vi "Configuration Utility.vi"() -> ()   [LabVIEW 2013, in "configuration library.lvlib"]
doc: "This is the main VI for the configuration editor."
uses:
  configuration library.lvlib
  Controls/StateCluster.ctl
  <vilib>/NI/Tag Bus Data Framework/Configuration Editor/Classes/SystemConfigRepo/SystemConfigRepo.lvclass
  <vilib>/NI/Configuration Framework/Node/NodeRef.ctl
  <vilib>/NI/Configuration Framework/Node/NISE_CEF_Node.lvclass
  subVI/SplashScreen/splash screen.ctl
  subVI/SplashScreen/notifier data.ctl
  <vilib>/NI/Configuration Framework/Node/StandardEvents.ctl
  <vilib>/NI/Configuration Framework/Node/UserEventRef.ctl
  <vilib>/NI/Configuration Framework/Controls/EventCluster.ctl
  <vilib>/NI/Configuration Framework/Node/NodeChangeEvent.ctl
  <vilib>/NI/Configuration Framework/Node/CacheState.ctl
  <vilib>/NI/Configuration Framework/Node/RefreshUIEvent.ctl
  <vilib>/NI/Configuration Framework/Node/StopEvent.ctl
  <vilib>/NI/Configuration Framework/glyph manager/glyph manager.ctl
  <vilib>/picture/picture.llb/imagedata.ctl
  Controls/add message.ctl
  Controls/MoveMessage.ctl
  <vilib>/NI/Tag Bus Data Framework/Configuration Editor/Classes/Systems/Systems.lvclass
  <vilib>/NI/Configuration Framework/Repository/NISE_CEF_Repository.lvclass
  <vilib>/NI/AMC/Create Single Message.vi
  <vilib>/NI/AMC/Update Message Routing Info.vi
  <vilib>/NI/AMC/Read Termination Message.vi
  <vilib>/NI/Tag Bus Data Framework/Configuration Editor/subVIs/Glyphs Status.ctl
  <vilib>/NI/Tag Bus Data Framework/Configuration Editor/subVIs/Add status to name.vi
  <vilib>/NI/AMC/Send Message.vi
  <vilib>/NI/AMC/Globals.vi
  <vilib>/NI/Tag Bus Data Framework/Configuration Editor/Classes/Module editor node/module editor node.lvclass
  <vilib>/NI/Tag Bus Data Framework/Configuration Editor/Classes/EngineTags/EngineTags.lvclass
  <vilib>/NI/Module Timing Source/timing source/TBM timing source.lvclass
  <vilib>/NI/Tag Bus Data Framework/Configuration Editor/Classes/TBM Configuration Node/TBM Configuration Node.lvclass
  <vilib>/NI/Tag Bus Module Framework/root configuration/TBM configuration.lvclass
  <vilib>/NI/Tag Bus Data Framework/Framework Configuration Classes/target configuration/PL_Target Configuration.lvclass
  <vilib>/NI/Tag Bus Data Framework/Configuration Editor/Classes/Targets/Targets.lvclass
  <vilib>/NI/Tag Bus Data Framework/Configuration Editor/Classes/Engine Parent/Engine Parent Editor Node.lvclass
  <vilib>/NI/Tag Bus Data Framework/Framework Configuration Classes/system configuration/PL_System Configuration.lvclass
  <vilib>/NI/Module Execution Interface/Engine Configuration/engine configuration.lvclass
  <vilib>/NI/Tag Bus Module Framework/channel/TBM channel.lvclass
  <vilib>/NI/Tag Bus Module Framework/module configuration/TBM module configuration.lvclass
  <vilib>/NI/AMC/AMC.lvlib
  <vilib>/NI/Configuration Framework/NISE_CEF_TreeControl.lvlib
  subVI/SplashScreen/splash screen.lvlib
  <vilib>/NI/Tag Bus Data Framework/Framework Configuration Classes/class cache/PL_class cache.lvlib
  <vilib>/NI/Tag Bus Data Framework/Configuration Editor/PL Framework Configuration Tool.lvlib
  <vilib>/NI/Configuration Framework/hierarchy repo/NISE_CEF_HierarchyRepo.lvclass
  <vilib>/NI/Configuration Framework/tree serializer/NISE_CEF_TreeSerializer.lvlib
  <vilib>/NI/Configuration Framework/glyph manager/glyph manager.lvlib
panel:
  in  "Exit":bool
  in  "View":string(tree)
  # "Tag Bus Configuration Editor"
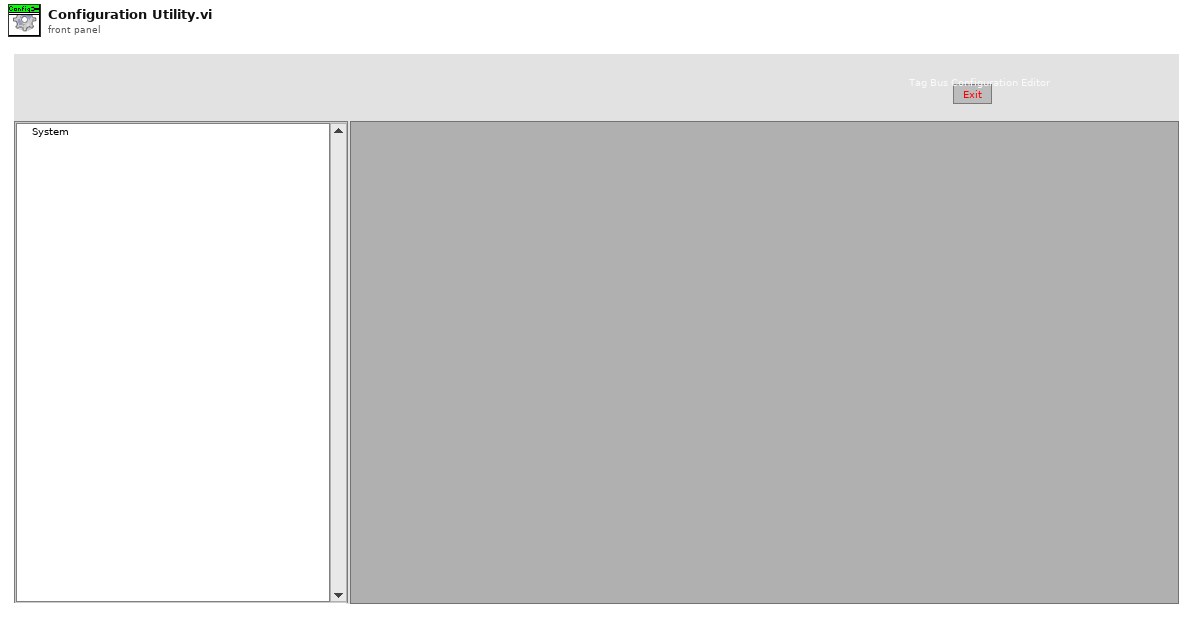
[diagram p1: front panel]
types:
  T1 = enum32{"Invalid", "Standard", "Closed", "Hidden", "Minimized", "Maximized"}
  T2 = typedef "configuration library.lvlib/StateCluster.ctl" = cluster{"repository":refnum<class "SystemConfigRepo.lvclass">, "root":T3, "unsaved changes":bool, "current path":path, "SplashScreen":T4, "classes cache":path, "standard events":T5, "glyph manager":T11}
  T3 = typedef "NISE_CEF_Node.lvclass/NodeRef.ctl" = refnum<data-value>
  T4 = typedef "configuration library.lvlib/splash screen.lvlib/splash screen.ctl" = cluster{"reference":refnum<vi>, "update notifier":refnum<notifier>, "Initialized":bool}
  T5 = typedef "NISE_CEF_Node.lvclass/StandardEvents.ctl" = cluster{"user event":T6, "node change":T7, "cache state":T8, "refresh UI":T9, "stop event":T10}
  T6 = typedef "NISE_CEF_Node.lvclass/UserEventRef.ctl" = refnum<user-event>
  T7 = typedef "NISE_CEF_Node.lvclass/NodeChangeEvent.ctl" = refnum<user-event>
  T8 = typedef "NISE_CEF_Node.lvclass/CacheState.ctl" = refnum<user-event>
  T9 = typedef "NISE_CEF_Node.lvclass/RefreshUIEvent.ctl" = refnum<user-event>
  T10 = typedef "NISE_CEF_Node.lvclass/StopEvent.ctl" = refnum<user-event>
  T11 = typedef "glyph manager.lvlib/glyph manager.ctl" = cluster{"search paths":path[], "glyph map":variant, "base glyphs":T12[], "desired overlays":string[]}
  T12 = typedef "imagedata.ctl" = cluster{"image type":i32, "image depth":i32, "image":u8[], "mask":u8[], "colors":u32[], "Rectangle":cluster{"left":i16, "top":i16, "right":i16, "bottom":i16}}
  T13 = typedef "AMC.lvlib/Message Queue.ctl" = refnum<queue>
  T14 = typedef "configuration library.lvlib/splash screen.lvlib/notifier data.ctl" = cluster{"Text":string, "percent":dbl}
  T15 = cluster{"node id":string, "RightClickPath":string}
  T16 = typedef "configuration library.lvlib/add message.ctl" = cluster{"node type":string, "to add to":string}
  T17 = typedef "configuration library.lvlib/MoveMessage.ctl" = cluster{"node ref":T3, "new parent":T3}
  T18 = typedef "configuration library.lvlib/FilePaths.ctl" = cluster{"glyphs":path[], "classes":path, "classes cache":path}
  T19 = typedef "PL_class cache.lvlib/cache definition.ctl" = cluster{"configuration":T20, "class cache data":T21}
  T20 = typedef "PL_class cache.lvlib/cache search configuration.ctl" = cluster{"Search Paths":path[], "Folders to Exclude":string[], "full class list":path[]}
  T21 = typedef "PL_class cache.lvlib/cached class information.ctl" = cluster{"targets":T22[], "engines":T23[], "modules":T23[], "ignored class list":path[]}
  T22 = typedef "PL_class cache.lvlib/target class metadata.ctl" = cluster{"file name":string, "fully qualified name":string, "menu display name":string, "configuration class name":string}
  T23 = typedef "PL_class cache.lvlib/class metadata.ctl" = cluster{"file name":string, "fully qualified name":string, "menu display name":string, "configuration class":string, "instances allowed":i32, "supported targets":T24[]}
  T24 = typedef "TBM configuration.lvclass/Target Types.ctl" = enum16{"Windows", "Mac", "Linux", "Linux RT ARM", "VxWorks", "Pharlap", "Other", "Linux RT x64"}
  T25 = typedef "NISE_CEF_Node.lvclass/Summary.ctl" = cluster{"ID":string, "parent ID":string, "node type":string, "text":string, "additional text":string, "glyph":string, "depth":i32, "glyph overlay":string}
  T26 = typedef "LVPoint32TypeDef.ctl" = cluster{"Horizontal":i32, "Vertical":i32}
  T27 = cluster{"data name":string, "drag data":variant}[]
  T28 = typedef "NISE_CEF_Node.lvclass/NodeMenuOptions.ctl" = cluster{"removable":bool, "movable":bool, "duplicate":bool}
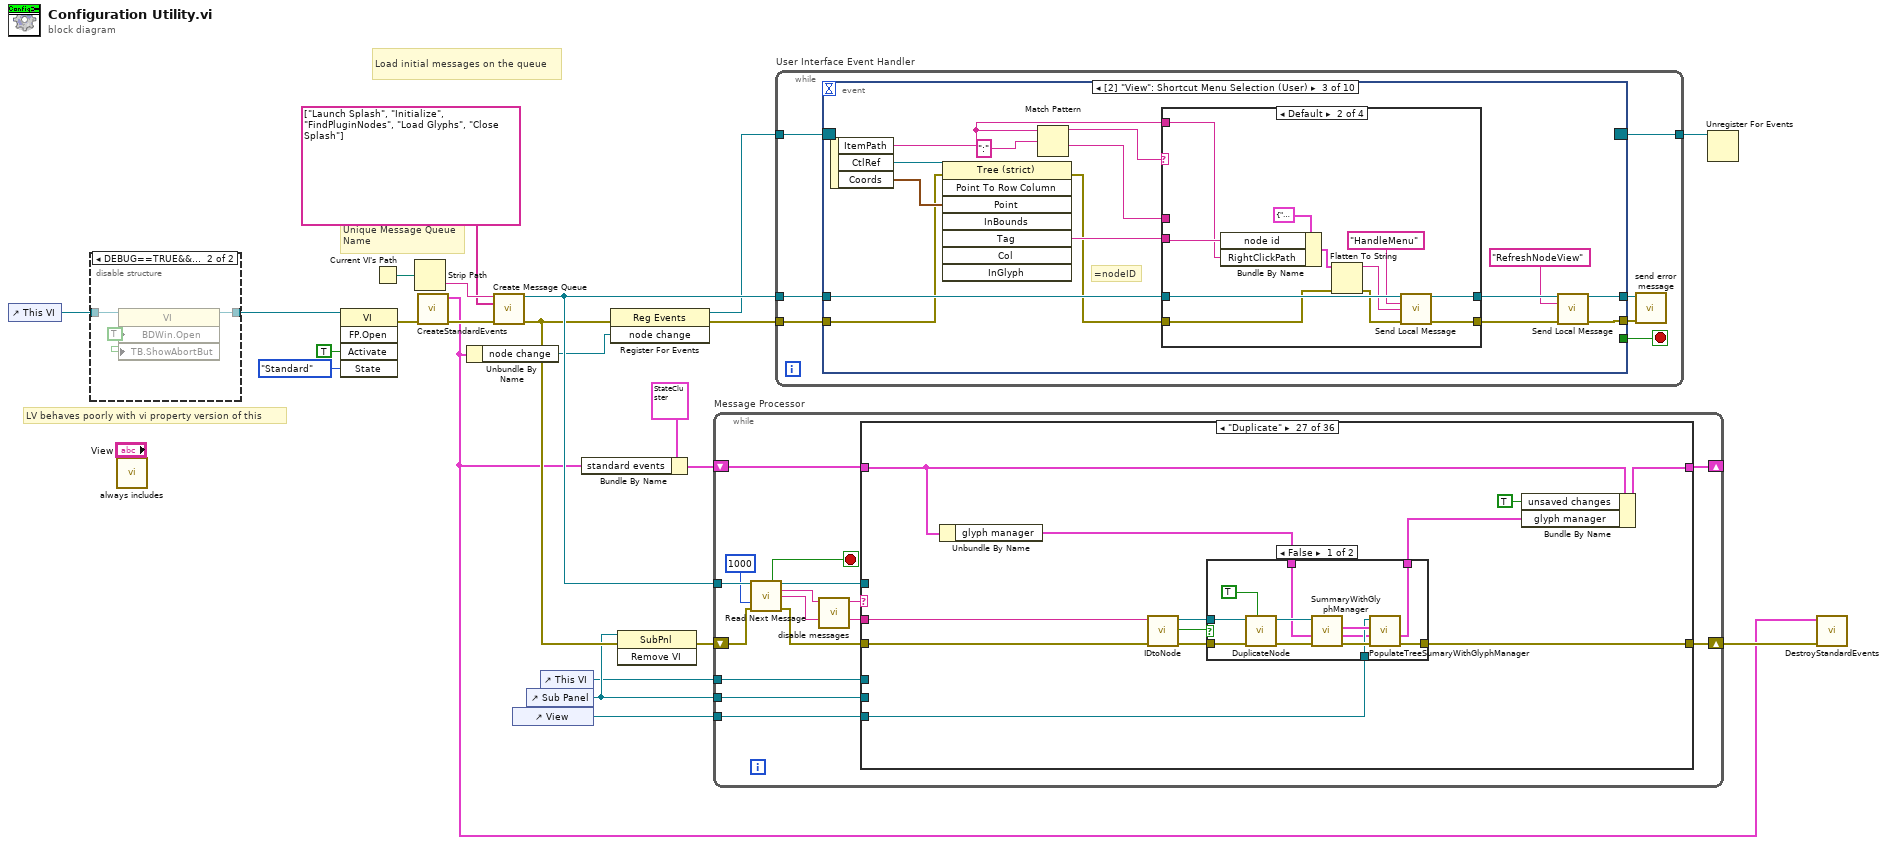
[diagram p0: block diagram]
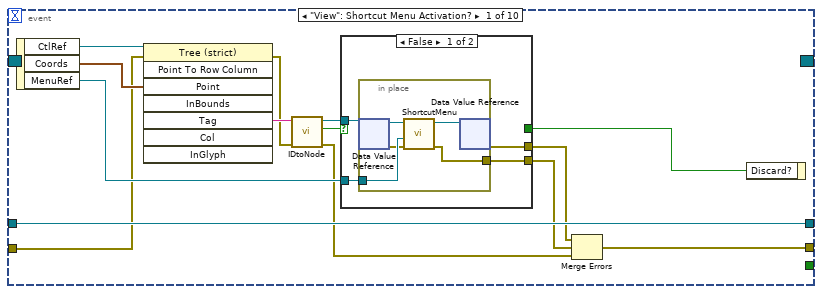
[diagram p3: hidden frame]
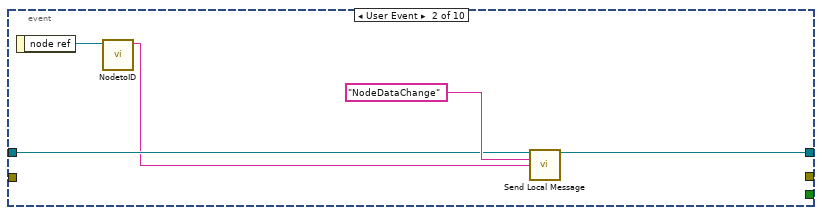
[diagram p5: hidden frame]
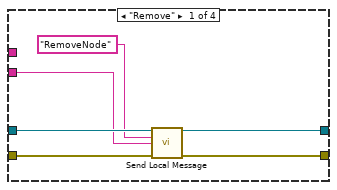
[diagram p6: hidden frame]
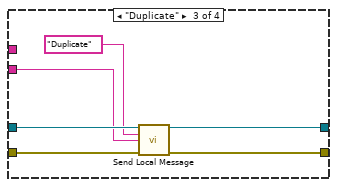
[diagram p7: hidden frame]
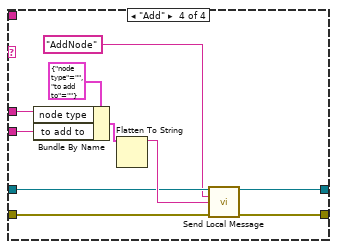
[diagram p8: hidden frame]
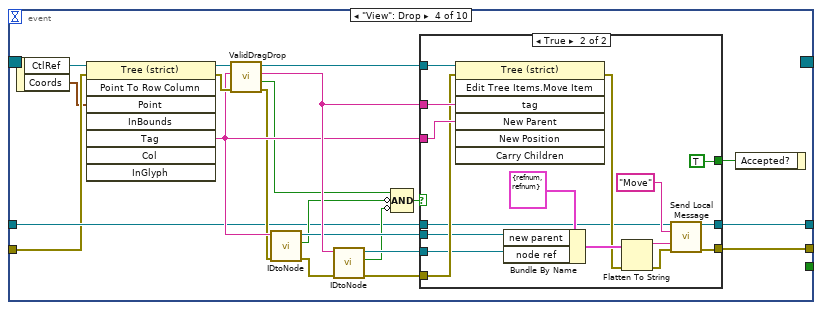
[diagram p9: hidden frame]
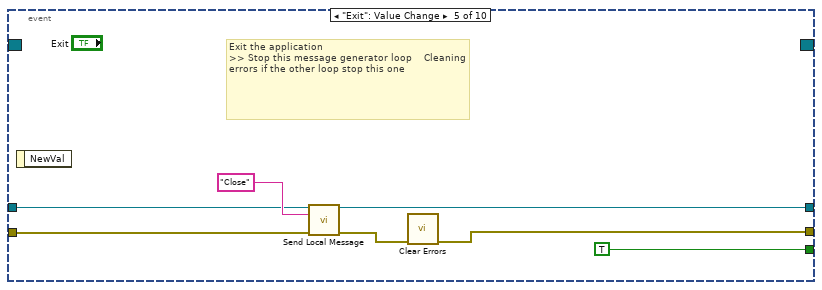
[diagram p11: hidden frame]
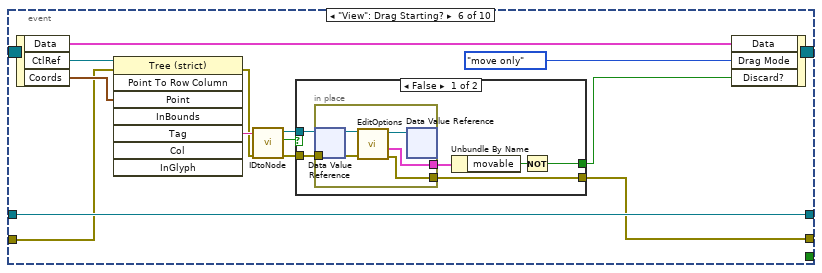
[diagram p12: hidden frame]
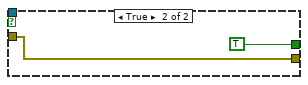
[diagram p13: hidden frame]
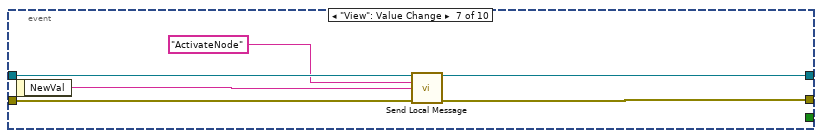
[diagram p14: hidden frame]
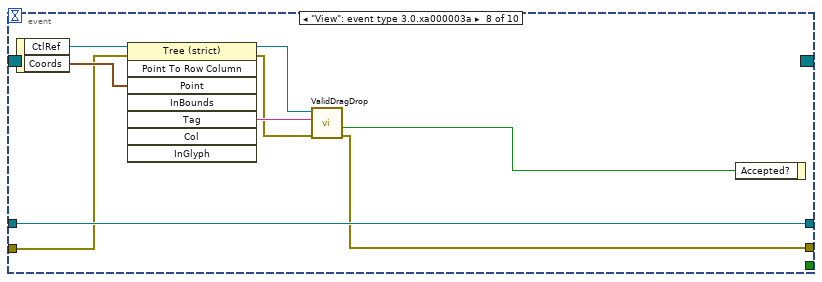
[diagram p15: hidden frame]
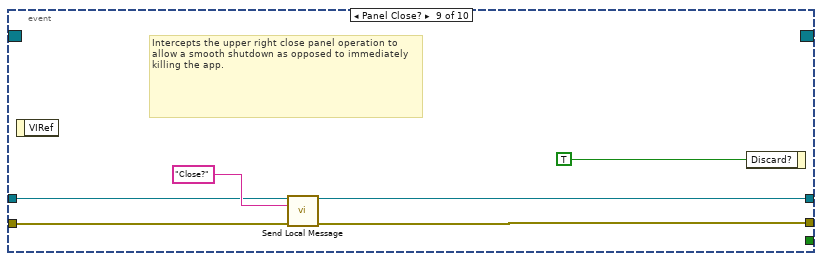
[diagram p16: hidden frame]
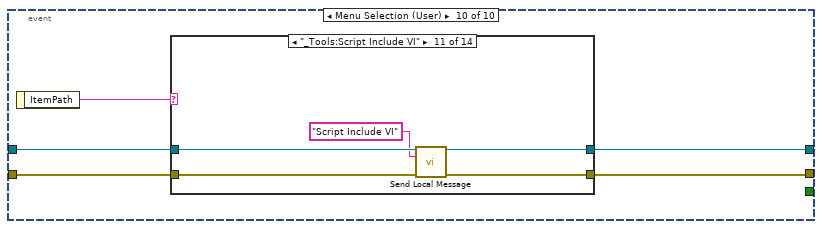
[diagram p17: hidden frame]
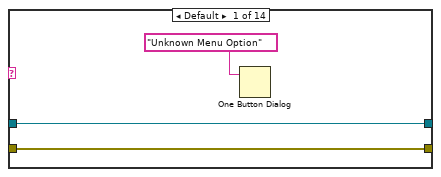
[diagram p18: hidden frame]
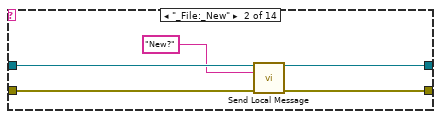
[diagram p19: hidden frame]
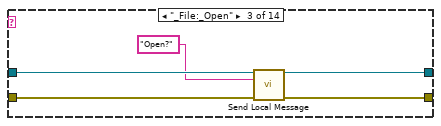
[diagram p20: hidden frame]
diagram:
  # "LV behaves poorly with vi property version of this"
  # "Unique Message Queue Name"
  # "Load initial messages on the queue"
  n1 = control-ref of="This VI"() -> (w14:refnum<vi>)
  n2 = disable-structure shown="DEBUG==TRUE&&RUN_TIME_ENGINE==False" {
    disable-tunnel: [w24 w27] -> w15
    disable-tunnel: w14 -> [w24 w26]
    frame condition #0 (active) {
    }
    frame condition #1 {
      w25 = TRUE ("Block Diagram Window:Open")
      n3 = property class="VI"(reference=w26, "BDWin.Open"=w25, "TB.ShowAbortBut"=w25) -> (reference out=w27:refnum<vi>)  [unwired: 1 in, 1 out]
    }
  }
  n4 = call "always includes.vi"() -> ()  [unwired: 12 in]
  n5 = invoke class="VI" method="FP.Open"(reference=w15, "Activate"=TRUE ("Activate?"), "State"=T1."Standard") -> (error out=w9:errorcluster)  [unwired: 2 in, 4 out]
  n6 = Current VI's Path() -> (path=w22:path)
  n7 = Strip Path(path=w22) -> (name=w23:string)  [unwired: 1 out]
  n8 = call <vilib>:"CreateStandardEvents.vi"("error in"=w9) -> ("error out"=w8:errorcluster, "standard events"=w1:T5)  [unwired: 9 in]
  n9 = Unbundle By Name(w1) -> ("node change"=w6:T7)
  n10 = call <vilib>:"Create Message Queue.vi"("message queue name"=w23, "initial message names"=string[] ["Launch Splash", "Initialize", "FindPluginNodes", "Load Glyphs", "Close Splash"], "error in"=w8) -> ("message queue out"=w20:T13, "error out"=w18:errorcluster)  [unwired: 11 in]
  n11 = control-ref of="View"() -> (w13:refnum<vi>)
  n12 = control-ref of="Sub Panel"() -> (w11:refnum<vi>)
  n13 = control-ref of="This VI"() -> (w10:refnum<vi>)
  n14 = Bundle By Name(cluster=T2 {"repository"=refnum, "root"=refnum, "unsaved changes"=FALSE, "current path"=path "", "SplashScreen"={"reference"=refnum, "update notifier"=refnum, "Initialized"=FALSE}, "classes cache"=path "", "standard events"={"user event"=refnum, "node change"=refnum, "cache state"=refnum, "refresh UI"=refnum, "stop event"=refnum}, "glyph manager"={"search paths"=[], "glyph map"=variant, "base glyphs"=[], "desired overlays"=[]}}, "standard events"=w1) -> (w4:T2)
  n15 = register-events(error in=w18, w6) -> (reference out=w5:refnum<event-registration>, error out=w7:errorcluster)  [unwired: 1 in]
  n16 = invoke class="SubPnl" method="Remove VI"(reference=w11, error in=w18) -> (error out=w12:errorcluster)  [unwired: 1 in, 2 out]
  n17 = while "Message Processor" {
    shift-right: [w40] -> w2
    shift-left: w12 -> [w39]
    tunnel: w20 -> [w38]
    shift-right: [w36] -> _
    shift-left: w4 -> [w35]
    tunnel: w10 -> [w30]
    tunnel: w11 -> [w29]
    tunnel: w13 -> [w28]
    stop <- w42 stop-if-true
    n18 = call <vilib>:"Read Next Message.vi"("message queue in"=w38, "timeout (1 ms)"=1000, "error in"=w39) -> ("exit process?"=w42:bool, "message queue out"=w34:T13, "message name"=w31:string, "message value"=w33:string, "error out"=w41:errorcluster)  [unwired: 5 in, 3 out]
    n19 = call "disable messages.vi"("message to check"=w31) -> ("message out"=w32:string)  [unwired: 10 in]
    n20 = case shown="\"Duplicate\"" w32 {
      selector: w32 -> [_ w46 _ _ _ _ _ _ _ _ _ w165 _ _ _ w288 _ _ _ _ _ _ _ _ _ _ _ _ _ _ _ _ _ _ _ _]
      tunnel: w33 -> [_ _ _ _ _ _ _ _ w121 _ _ _ _ _ _ _ _ w331 _ _ w400 _ w446 _ _ w498 w516 w539 _ w569 _ _ w624 w649 _ w658]
      tunnel: w41 -> [w44 w49 w51 w58 w71 w79 w106 w112 w122 w148 w152 w162 w189 w215 w250 w281 w308 w336 w353 w360 w398 w415 w447 w467 w470 w497 w515 w540 w555 w568 w602 w612 w623 w648 w655 w661]
      tunnel: [w44 w49 w51 w61 w68 w78 w107 w115 errorcluster {"status"=FALSE, "code"=0, "source"=""} ("error out") w146 w152 w167 w206 w208 w243 w291 w318 w335 w352 w362 w385 w414 w435 w466 w470 w479 w517 w542 w555 w567 w599 w610 w622 w647 w653 w660] -> w40
      tunnel: [w43 w45 w50 w59 w63 w77 w97 w113 w123 w145 w151 w163 w204 w207 w242 w292 w319 w332 w354 w361 w401 w411 w432 w468 w469 w482 w510 w541 w556 w559 w591 w611 w620 w638 w654 w657] -> w36
      tunnel: w35 -> [w43 w45 w50 w60 w72 w87 w98 w113 w123 w145 w151 w164 w188 w216 w251 w287 w314 w333 w354 w361 w401 w412 w433 w468 w469 w496 w508 w534 w557 w561 w607 w611 w620 w650 w654 w663]
      tunnel: w34 -> [_ _ _ _ _ _ w108 w114 w125 w147 _ w166 w205 w214 w249 w278 w317 w334 _ w363 _ w413 w437 _ _ _ _ _ _ _ _ _ w621 w646 _ w659]
      tunnel: w30 -> [_ _ _ w52 w67 _ w95 _ _ _ _ _ _ _ _ _ _ _ _ _ _ _ _ _ _ _ _ _ _ _ w598 _ _ _ _ _]
      tunnel: w29 -> [_ _ _ _ _ _ _ _ w117 w139 _ w154 _ _ _ w279 w306 _ _ _ _ _ _ _ _ _ _ _ _ w562 _ w609 w613 _ _ _]
      tunnel: w28 -> [_ _ _ _ _ w75 _ _ _ _ _ w153 _ _ _ _ _ _ _ _ _ _ w436 _ _ w483 w511 w535 _ w563 w601 _ _ _ _ _]
      frame "", "Idle" {
      }
      frame "Missing Message Handler", Default {
        # "Call this case if a message is received that is not handled by any other case. Typically this is a programming error as a result of a typo or unhandled message/missing message handler."
        n21 = Format Into String(format string="Internal Error: Missing message handler for '%s\" message." ("message"), w46) -> (resulting string=w48:string)  [unwired: 2 in, 1 out]
        n22 = One Button Dialog(message=w48) -> ()  [unwired: 2 out]
      }
      frame "------------Generic Operations------------" {
        # "Dummy case to add a seperation in the Case Structure menu"
      }
      frame "Launch Splash" {
        n23 = invoke class="VI" method="FP.Center"(reference=w52, error in=w58) -> (reference out=w56:refnum<vi>, error out=w55:errorcluster)  [unwired: 1 in, 1 out]
        n24 = invoke class="VI" method="FP.Open"(reference=w56, error in=w55, "State"=T1."Hidden") -> (error out=w53:errorcluster)  [unwired: 2 in, 4 out]
        n25 = call "Launch.vi"("error in"=w53) -> ("error out"=w61:errorcluster, "SplashScreen"=w57:T4)  [unwired: 9 in]
        n26 = Bundle By Name(cluster=w60, "SplashScreen"=w57) -> (w59:T2)
      }
      frame "Initialize" {
        # "issues in exe"
        n27 = Current VI's Menubar() -> (w70:refnum<k9>)
        n28 = call "menu options.vi"("error in"=w71, "VI ref"=w67, "menu ref in"=w70) -> ("error out"=w68:errorcluster)  [unwired: 7 in, 1 out]
        n29 = call "default file paths.vi"() -> ("paths"=w69:T18)  [unwired: 11 in]
        n30 = Unbundle By Name(w69) -> ("classes cache"=w66:path)
        n31 = Bundle By Name(cluster=w72, "classes cache"=w66) -> (w63:T2)
        n32 = Unbundle By Name(w63) -> ("SplashScreen"=w62:T4)
        n33 = call "Update.vi"("Update"=T14 {"Text"="Preparing UI...", "percent"=27.0}, "SplashScreen in"=w62) -> ("error out"=w65:errorcluster)  [unwired: 8 in, 1 out]
        n34 = call <vilib>:"Clear Errors.vi"("error in (no error)"=w65) -> ()  [unwired: 6 in, 1 out]
      }
      frame "Load Glyphs" {
        n35 = Unbundle By Name(w87) -> ("SplashScreen"=w86:T4)
        n36 = call "default file paths.vi"() -> ("paths"=w74:T18)  [unwired: 11 in]
        n37 = invoke class="Tree (strict)" method="Custom Item Symbols.Revert Symbols"(reference=w75, error in=w79) -> (reference out=w85:refnum<vi>, error out=w84:errorcluster)  [unwired: 1 in, 1 out]
        n38 = Unbundle By Name(w74) -> ("glyphs"=w73:path[])
        n39 = call <vilib>:"create glyph manager.vi"("error in"=w84, "tree ref (for default symbols)"=w85) -> ("error out"=w80:errorcluster, "glyph manager"=w81:T11)  [unwired: 8 in]
        n40 = call "Update.vi"("Update"=T14 {"Text"="Loading Glyphs...", "percent"=78.0}, "SplashScreen in"=w86) -> ("error out"=w89:errorcluster)  [unwired: 8 in, 1 out]
        n41 = for {
          tunnel: w73 -> [w90] mode=indexing
          shift-right: [w94] -> w83
          shift-left: w81 -> [w92]
          shift-right: [w93] -> w82
          shift-left: w80 -> [w91]
          n42 = call <vilib>:"add search path.vi"("error in"=w91, "search path"=w90, "glyph manager in"=w92) -> ("error out"=w93:errorcluster, "glyph manager out"=w94:T11)  [unwired: 7 in]
        }
        n43 = call <vilib>:"Clear Errors.vi"("error in (no error)"=w89) -> ()  [unwired: 6 in, 1 out]
        n44 = call <vilib>:"update tree control.vi"("error in"=w82, "tree reference"=w85, "glyph manager in"=w83) -> ("error out"=w78:errorcluster, "glyph manager out"=w76:T11)  [unwired: 7 in]
        n45 = Bundle By Name(cluster=w87, "glyph manager"=w76) -> (w77:T2)
      }
      frame "Close Splash" {
        n46 = Unbundle By Name(w98) -> ("SplashScreen"=w104:T4)
        n47 = call "Close.vi"("error in"=w106, "SplashScreen"=w104) -> ("error out"=w100:errorcluster, "SplashScreen out"=w96:T4)  [unwired: 8 in]
        n48 = Bundle By Name(cluster=w98, "SplashScreen"=w96) -> (w97:T2)
        n49 = invoke class="VI" method="FP.Open"(reference=w95, error in=w100, "State"=T1."Standard") -> (reference out=w102:refnum<vi>, error out=w101:errorcluster)  [unwired: 2 in, 3 out]
        n50 = Close Reference(reference=w102, error in (no error)=w101) -> (error out=w99:errorcluster)
        n51 = call <vilib>:"Send Local Message.vi"("message queue in"=w108, "message name"="New" ("Message Name"), "error in"=w99) -> ("error out"=w107:errorcluster)  [unwired: 10 in, 2 out]
      }
      frame "Close" {
        n52 = Unbundle By Name(w113) -> ("root"=w110:T3)
        n53 = call <vilib>:"CloseNode.vi"("error in"=w112, "node ref"=w110) -> ("error out"=w109:errorcluster)  [unwired: 9 in]
        n54 = call <vilib>:"Send Local Message.vi"("message queue in"=w114, "message name"="Exit", "error in"=w109) -> ("error out"=w115:errorcluster)  [unwired: 10 in, 2 out]
      }
      frame "Error" {
        n55 = Unbundle By Name(w123) -> ("standard events"=w116:T5)
        n56 = call "Remove UI without races.vi"("error in"=w122, "standard events"=w116, "sub panel ref in"=w117) -> ("error out"=w118:errorcluster)  [unwired: 7 in, 1 out]
        n57 = case shown="\"\"" w121 {
          selector: w121 -> [w127 _]
          tunnel: w122 -> [w128 w129]
          tunnel: [w126 w129] -> w119
          frame Default {
            n58 = Unflatten From String(type=w128, binary string=w127, error in (no error)=w128) -> (value=w126:errorcluster)  [unwired: 2 in, 2 out]
          }
          frame "" {
          }
        }
        n59 = call <vilib>:"Clear Errors.vi"("error in (no error)"=w118) -> ()  [unwired: 6 in, 1 out]
        n60 = Unbundle By Name(w119) -> ("code"=w120:i32)
        n61 = case shown="15550" w120 {
          tunnel: w125 -> [_ _ _ w135 _]
          tunnel: w119 -> [_ _ _ w134 w137]
          frame -2147220623, -2147220621, -2147220364, 56, 63 {
            n62 = One Button Dialog(message="Problem communicating with remote device.  Make sure a valid device is selected and that the IP address is correct.") -> ()  [unwired: 1 in, 1 out]
          }
          frame 1003 {
            n63 = One Button Dialog(message="Dev Error: The Ui.vi for the selected class is broken") -> ()  [unwired: 1 in, 1 out]
          }
          frame 15550 {
            n64 = One Button Dialog(message="The cRIO does not yet have a configuration to download. Create or open a configuration and download it to the cRIO") -> ()  [unwired: 1 in, 1 out]
          }
          frame 537549 {
            n65 = call <vilib>:"Send Local Message.vi"("message queue in"=w135, "message name"="Exit", "error in"=w134) -> ()  [unwired: 10 in, 3 out]
            n66 = One Button Dialog(message="Invalid configuration file.") -> ()  [unwired: 1 in, 1 out]
          }
          frame 1, Default {
            n67 = call <vilib>:"Simple Error Handler.vi"("error in (no error)"=w137) -> ()  [unwired: 1 in, 8 out]
          }
        }
      }
      frame "Exit" {
        # "Stop the VI                                                                             >> Perform any cleanup tasks in this message case. >> Clear display before closing."
        n68 = call <vilib>:"Destroy Message Queue.vi"("message queue in"=w147, "error in"=w148) -> ("error out"=w142:errorcluster)  [unwired: 11 in, 2 out]
        n69 = control-ref of="Exit"() -> (w144:refnum<vi>)
        n70 = Unbundle By Name(w145) -> ("standard events"=w138:T5)
        n71 = property class="Bool (strict)"(reference=w144, error in=w142, "Val(Sgnl)"=FALSE ("Exit")) -> (error out=w141:errorcluster)  [unwired: 1 out]
        n72 = call "Remove UI without races.vi"("error in"=w141, "standard events"=w138, "sub panel ref in"=w139) -> ("error out"=w140:errorcluster)  [unwired: 7 in, 1 out]
        n73 = disable-structure shown="RUN_TIME_ENGINE==True" {
          disable-tunnel: [w149 w150] -> w146
          disable-tunnel: w140 -> [w149 w150]
          frame condition #0 (active) {
          }
          frame condition #1 {
            n74 = Quit LabVIEW() -> ()  [unwired: 1 in]
          }
        }
      }
      frame "------------Menu Operations--------------" {
        # "Dummy case to add a seperation in the Case Structure menu"
      }
      frame "Close?", "New?", "Open?" {
        n75 = Unbundle By Name(w164) -> ("unsaved changes"=w155:bool, "standard events"=w156:T5)
        n76 = case shown="True" w155 {
          tunnel: [TRUE ("SaveFlag") w185] -> w158
          tunnel: w164 -> [w177 w184]
          tunnel: [w177 w183] -> w163
          tunnel: w162 -> [w176 w182]
          tunnel: [w176 w181] -> w157
          tunnel: w154 -> [_ w180]
          tunnel: w153 -> [_ w179]
          frame False {
            # "If there is nothing to save Go do Action"
          }
          frame True {
            n77 = call "dialog save dirty dot.vi"("error in"=w182, "View"=w179, "sub panel ref in"=w180, "state in"=w184) -> ("error out"=w181:errorcluster, "new"=w185:bool, "state out"=w183:T2)  [unwired: 5 in]
          }
        }
        n78 = Search and Replace String(input string=w165, search string="?", replace string="") -> (result string=w159:string)  [unwired: 5 in, 3 out]
        n79 = case shown="True" w158 {
          tunnel: w157 -> [w168 w175]
          tunnel: [w168 w171] -> w167
          tunnel: w166 -> [_ w174]
          tunnel: w159 -> [_ w173]
          tunnel: w156 -> [_ w169]
          tunnel: w154 -> [_ w170]
          frame False {
          }
          frame True {
            n80 = call <vilib>:"Send Local Message.vi"("message queue in"=w174, "message name"=w173, "error in"=w175) -> ("error out"=w172:errorcluster)  [unwired: 10 in, 2 out]
            n81 = call "Remove UI without races.vi"("error in"=w172, "standard events"=w169, "sub panel ref in"=w170) -> ("error out"=w171:errorcluster)  [unwired: 7 in, 1 out]
          }
        }
      }
      frame "New" {
        # "unused"
        n82 = Unbundle By Name(w188) -> ("glyph manager"=w187:T11)
        n83 = call <vilib>:"create default cache.vi"() -> ("cache"=w195:T19)  [unwired: 11 in]
        n84 = Unbundle By Name(w195) -> ("configuration.Search Paths"=w194:path[])
        n85 = call-dynamic "AddGlyphtoGManager.vi"("error in"=w189, "glyph manager"=w187, "NISE_CEF_serializable node in"=refnum<class "Systems.lvclass"> refnum ("Systems.lvclass")) -> ("error out"=w190:errorcluster, "glyph manager out"=w186:T11, "NISE_CEF_serializable node out"=w191:refnum<class "Systems.lvclass">)  [unwired: 6 in]
        n86 = call-dynamic "Initialize.vi"("error in"=w190, "node in"=w191) -> ("error out"=w200:errorcluster, "data value reference"=w201:T3)  [unwired: 7 in, 1 out]
        n87 = Delete From Array(array=w194) -> (deleted portion=w193:path)  [unwired: 2 in, 1 out]
        n88 = call-dynamic "Initialize.vi"("error in"=w200, "path"=w193, "repository in"=refnum<class "SystemConfigRepo.lvclass"> refnum ("SystemConfigRepo.lvclass")) -> ("error out"=w199:errorcluster, "repository out"=w198:refnum<class "SystemConfigRepo.lvclass">)  [unwired: 7 in]
        n89 = Bundle By Name(cluster=w188, "unsaved changes"=FALSE ("SaveFlag"), "repository"=w198, "root"=w201, "current path"=path "", "glyph manager"=w186) -> (w204:T2)
        n90 = call <vilib>:"Send Local Message.vi"("message queue in"=w205, "message name"="PopulateTree", "error in"=w199) -> ("error out"=w206:errorcluster)  [unwired: 10 in, 2 out]
      }
      frame "Open" {
        n91 = call <vilib>:"Set Busy.vi"() -> ("error out"=w211:errorcluster)  [unwired: 10 in, 1 out]
        n92 = call "File Dialog"("pattern (all files)"="*.pcfg") -> ("selected path"=w213:path, "cancelled"=w212:bool)  [unwired: 11 in, 2 out]
        n93 = case shown="False" w212 {
          tunnel: w216 -> [w225 w241]
          tunnel: [w224 w241] -> w207
          tunnel: w215 -> [w223 w240]
          tunnel: w214 -> [w222 _]
          tunnel: [w221 w240] -> w208
          tunnel: w213 -> [w218 _]
          tunnel: w211 -> [w217 w239]
          tunnel: [w217 w239] -> w210
          frame False {
            n94 = in-place {
              in-place-border: w223 -> [w238]
              in-place-border: [w227] -> w219
              in-place-border: w218 -> [w233]
              n95 = in-place-cluster #1(w225) -> ("repository"=w226:refnum<class "SystemConfigRepo.lvclass">, "current path"=w234:path)  [unwired: 2 out]
              n96 = call-dynamic "Open.vi"("error in"=w238, "file path"=w233, "repository in"=w226) -> ("error out"=w235:errorcluster, "repository out"=w231:refnum<class "SystemConfigRepo.lvclass">)  [unwired: 6 in, 1 out]
              n97 = call-dynamic "WriteTree.vi"("error in"=w235, "repository in"=w231) -> ("error out"=w228:errorcluster, "root"=w236:T3, "repository out"=w230:refnum<class "NISE_CEF_Repository.lvclass">)  [unwired: 7 in]
              n98 = To More Specific Class(target class=w226, reference=w230, error in=w228) -> (specific class reference=w229:refnum<class "SystemConfigRepo.lvclass">, error out=w227:errorcluster)
              n99 = Select(t=w234, s=w227, f=w233) -> (s? t:f=w232:path)
              n100 = in-place-cluster #1("unsaved changes"=FALSE ("SaveFlag"), "repository"=w229, "root"=w236, "current path"=w232) -> (w224:T2)
            }
            n101 = call <vilib>:"Send Local Message.vi"("message queue in"=w222, "message name"="PopulateTree", "error in"=w219) -> ("error out"=w221:errorcluster)  [unwired: 10 in, 2 out]
          }
          frame True {
          }
        }
        n102 = call <vilib>:"Unset Busy.vi"("error in (no error)"=w210) -> ()  [unwired: 10 in, 1 out]
      }
      frame "Load Binary" {
        n103 = call <vilib>:"Set Busy.vi"() -> ("error out"=w246:errorcluster)  [unwired: 10 in, 1 out]
        n104 = call "File Dialog2"("pattern (all files)"="*.pbin") -> ("selected path"=w248:path, "cancelled"=w247:bool)  [unwired: 11 in, 2 out]
        n105 = case shown="False" w247 {
          tunnel: w251 -> [w260 w276]
          tunnel: [w259 w276] -> w242
          tunnel: w250 -> [w258 w275]
          tunnel: w249 -> [w257 _]
          tunnel: [w256 w275] -> w243
          tunnel: w248 -> [w253 _]
          tunnel: w246 -> [w252 w274]
          tunnel: [w252 w274] -> w245
          frame False {
            n106 = in-place {
              in-place-border: w258 -> [w263]
              in-place-border: [w268] -> w254
              in-place-border: w253 -> [w264]
              n107 = in-place-cluster #2(w260) -> ("repository"=w265:refnum<class "SystemConfigRepo.lvclass">)  [unwired: 2 out]
              n108 = call <vilib>:"read full file.vi"("error in"=w263, "file path"=w264) -> ("error out"=w262:errorcluster, "data"=w261:string)  [unwired: 8 in]
              n109 = call <vilib>:"unflatten memory.vi"("error in"=w262, "binary repo"=w261, "NISE_CEF_HierarchyRepo in"=w265) -> ("error out"=w266:errorcluster, "NISE_CEF_HierarchyRepo out"=w267:refnum<class "SystemConfigRepo.lvclass">)  [unwired: 7 in]
              n110 = call-dynamic "WriteTree.vi"("error in"=w266, "repository in"=w267) -> ("error out"=w269:errorcluster, "root"=w272:T3, "repository out"=w271:refnum<class "NISE_CEF_Repository.lvclass">)  [unwired: 7 in]
              n111 = To More Specific Class(target class=w265, reference=w271, error in=w269) -> (specific class reference=w270:refnum<class "SystemConfigRepo.lvclass">, error out=w268:errorcluster)
              n112 = in-place-cluster #2("unsaved changes"=TRUE ("SaveFlag"), "repository"=w270, "root"=w272) -> (w259:T2)
            }
            n113 = call <vilib>:"Send Local Message.vi"("message queue in"=w257, "message name"="PopulateTree", "error in"=w254) -> ("error out"=w256:errorcluster)  [unwired: 10 in, 2 out]
          }
          frame True {
          }
        }
        n114 = call <vilib>:"Unset Busy.vi"("error in (no error)"=w245) -> ()  [unwired: 10 in, 1 out]
      }
      frame "Save", "SaveAs" {
        n115 = Unbundle By Name(w287) -> ("standard events"=w277:T5)
        n116 = call <vilib>:"Set Busy.vi"() -> ("error out"=w285:errorcluster)  [unwired: 10 in, 1 out]
        n117 = call "Remove UI without races.vi"("error in"=w281, "standard events"=w277, "sub panel ref in"=w279) -> ("error out"=w280:errorcluster)  [unwired: 7 in, 1 out]
        n118 = flat-sequence {
          tunnel: w280 -> [w299]
          tunnel: w288 -> [w297]
          tunnel: w287 -> [w294]
          tunnel: w285 -> [w293]
          tunnel: [w300] -> w284
          tunnel: [w298] -> w283
          tunnel: [w293] -> w282
          tunnel: [w302] -> w286
          tunnel: [w303] -> w289
          tunnel: [w304] -> w292
          tunnel: w284 -> [w304]
          tunnel: w283 -> [w303]
          tunnel: w282 -> [w302]
          frame #0 {
            n119 = Equal?(x="SaveAs", y=w297) -> (x = y?=w296:bool)
            n120 = call "save operation.vi"("force save as"=w296, "error in"=w299, "state cluster"=w294) -> ("error out"=w298:errorcluster, "state out"=w300:T2)  [unwired: 7 in]
          }
          frame #1 {
            n121 = local read "View"() -> (w301:string)
            n122 = property on="View" class="Tree (strict)"("Val(Sgnl)"=w301) -> ()  [unwired: 2 in, 2 out]
          }
        }
        n123 = call <vilib>:"Unset Busy.vi"("error in (no error)"=w286) -> ()  [unwired: 10 in, 1 out]
        n124 = call <vilib>:"Send Local Message.vi"("message queue in"=w278, "message name"="PopulateTree", "error in"=w289) -> ("error out"=w291:errorcluster)  [unwired: 10 in, 2 out]
      }
      frame "Save Binary" {
        n125 = Unbundle By Name(w314) -> ("standard events"=w305:T5)
        n126 = call <vilib>:"Set Busy.vi"() -> ("error out"=w312:errorcluster)  [unwired: 10 in, 1 out]
        n127 = call "Remove UI without races.vi"("error in"=w308, "standard events"=w305, "sub panel ref in"=w306) -> ("error out"=w307:errorcluster)  [unwired: 7 in, 1 out]
        n128 = flat-sequence {
          tunnel: w307 -> [w323]
          tunnel: w314 -> [w320]
          tunnel: w312 -> [w324]
          tunnel: [w321] -> w311
          tunnel: [w322] -> w310
          tunnel: [w324] -> w309
          tunnel: [w326] -> w313
          tunnel: [w327] -> w315
          tunnel: [w328] -> w319
          tunnel: w311 -> [w328]
          tunnel: w310 -> [w327]
          tunnel: w309 -> [w326]
          frame #0 {
            n129 = call "save operation binary.vi"("error in"=w323, "state cluster"=w320) -> ("error out"=w322:errorcluster, "state out"=w321:T2)  [unwired: 8 in]
          }
          frame #1 {
            n130 = local read "View"() -> (w325:string)
            n131 = property on="View" class="Tree (strict)"("Val(Sgnl)"=w325) -> ()  [unwired: 2 in, 2 out]
          }
        }
        n132 = call <vilib>:"Unset Busy.vi"("error in (no error)"=w313) -> ()  [unwired: 10 in, 1 out]
        n133 = call <vilib>:"Send Local Message.vi"("message queue in"=w317, "message name"="PopulateTree", "error in"=w315) -> ("error out"=w318:errorcluster)  [unwired: 10 in, 2 out]
      }
      frame "Custom View" {
        n134 = in-place {
          in-place-border: w336 -> [w349]
          in-place-border: [w340] -> w329
          in-place-border: w331 -> [w341]
          n135 = in-place-cluster #3(w333) -> ("repository"=w338:refnum<class "SystemConfigRepo.lvclass">, "root"=w347:T3)
          n136 = call-dynamic "ReadTree.vi"("error in"=w349, "root"=w347, "repository in"=w338) -> ("error out"=w345:errorcluster, "repository out"=w343:refnum<class "NISE_CEF_Repository.lvclass">)  [unwired: 7 in]
          n137 = call-dynamic "CustomView.vi"("error in"=w345, "view name"=w341, "repository in"=w343) -> ("error out"=w344:errorcluster, "repository out"=w342:refnum<class "NISE_CEF_Repository.lvclass">)  [unwired: 7 in]
          n138 = call-dynamic "WriteTree.vi"("error in"=w344, "repository in"=w342) -> ("error out"=w348:errorcluster, "root"=w346:T3, "repository out"=w339:refnum<class "NISE_CEF_Repository.lvclass">)  [unwired: 7 in]
          n139 = To More Specific Class(target class=w338, reference=w339, error in=w348) -> (specific class reference=w337:refnum<class "SystemConfigRepo.lvclass">, error out=w340:errorcluster)
          n140 = in-place-cluster #3("repository"=w337, "root"=w346) -> (w332:T2)
        }
        n141 = call <vilib>:"Send Local Message.vi"("message queue in"=w334, "message name"="PopulateTree", "error in"=w329) -> ("error out"=w335:errorcluster)  [unwired: 10 in, 2 out]
      }
      frame "DeployTool" {
        n142 = Unbundle By Name(w354) -> ("current path"=w350:path, "root"=w351:T3)
        n143 = call <vilib>:"deployment tool.vi"("current pcfg path"=w350, "error in"=w353, "root"=w351) -> ("error out"=w352:errorcluster)  [unwired: 8 in]
      }
      frame "Edit Plugin Search Paths" {
        n144 = Unbundle By Name(w361) -> ("classes cache"=w359:path)
        n145 = call <vilib>:"load cache.vi"("error in"=w360, "cache path"=w359) -> ("error out"=w358:errorcluster, "cache"=w356:T19)  [unwired: 8 in]
        n146 = case shown="No Error" w358 {
          selector: w358 -> [w368 w371]
          tunnel: [w369 w372] -> w357
          tunnel: w356 -> [w369 _]
          tunnel: [w368 w370] -> w355
          frame No Error {
          }
          frame Error {
            n147 = call <vilib>:"create default cache.vi"() -> ("cache"=w372:T19)  [unwired: 11 in]
            n148 = call <vilib>:"Clear Errors.vi"("error in (no error)"=w371) -> ("error out"=w370:errorcluster)  [unwired: 6 in]
          }
        }
        n149 = Unbundle By Name(w357) -> ("configuration.Search Paths"=w367:path[])
        n150 = call "dialog edit search paths.vi"("error in"=w355, "Plugin Search Paths"=w367) -> ("error out"=w364:errorcluster, "Cancelled?"=w366:bool, "Plugin Search Paths"=w365:path[])  [unwired: 7 in]
        n151 = case shown="False" w366 {
          tunnel: w357 -> [w382 _]
          tunnel: w365 -> [w381 _]
          tunnel: w364 -> [w375 w383]
          tunnel: w363 -> [w378 _]
          tunnel: [w377 w383] -> w362
          tunnel: w359 -> [w373 _]
          frame False {
            n152 = Bundle By Name(cluster=w382, "configuration.Search Paths"=w381) -> (w374:T19)
            n153 = call <vilib>:"save cache.vi"("error in"=w375, "cache"=w374, "path"=w373) -> ("error out"=w376:errorcluster)  [unwired: 8 in]
            n154 = call <vilib>:"Send Local Message.vi"("message queue in"=w378, "message name"="FindPluginNodes", "message value"="Refresh", "error in"=w376) -> ("error out"=w377:errorcluster)  [unwired: 9 in, 2 out]
          }
          frame True {
          }
        }
      }
      frame "FindPluginNodes" {
        n155 = Unbundle By Name(w401) -> ("SplashScreen"=w391:T4, "classes cache"=w387:path)
        n156 = flat-sequence {
          tunnel: w398 -> [w402]
          tunnel: [w402] -> w397
          frame #0 {
            n157 = call <vilib>:"Set Busy.vi"() -> ()  [unwired: 10 in, 2 out]
          }
        }
        n158 = Equal?(x="Refresh", y=w400) -> (x = y?=w392:bool)
        n159 = call <vilib>:"load cache.vi"("error in"=w397, "cache path"=w387) -> ("error out"=w396:errorcluster, "cache"=w395:T19)  [unwired: 8 in]
        n160 = case shown="No Error" w396 {
          selector: w396 -> [w406 w407]
          tunnel: [w404 w408] -> w393
          tunnel: w395 -> [w405 _]
          tunnel: [w406 _] -> w394
          frame No Error {
            n161 = call <vilib>:"remove missing files.vi"("cache in"=w405) -> ("cache out"=w404:T19)  [unwired: 10 in]
          }
          frame Error {
            n162 = call <vilib>:"create default cache.vi"() -> ("cache"=w408:T19)  [unwired: 11 in]
            n163 = call <vilib>:"Clear Errors.vi"("error in (no error)"=w407) -> ()  [unwired: 6 in, 1 out]
          }
        }
        n164 = call <vilib>:"identify new classes.vi"("error in"=w394, "force scan"=w392, "cache in"=w393) -> ("error out"=w388:errorcluster, "cache out"=w384:T19)  [unwired: 7 in]
        n165 = call "Update.vi"("Update"=T14 {"Text"="Loading Classes...", "percent"=45.0}, "SplashScreen in"=w391) -> ("error out"=w390:errorcluster)  [unwired: 8 in, 1 out]
        n166 = call <vilib>:"Clear Errors.vi"("error in (no error)"=w390) -> ()  [unwired: 6 in, 1 out]
        n167 = call <vilib>:"save cache.vi"("error in"=w388, "cache"=w384, "path"=w387) -> ("error out"=w386:errorcluster)  [unwired: 8 in]
        n168 = flat-sequence {
          tunnel: w386 -> [w403]
          tunnel: [w403] -> w385
          frame #0 {
            n169 = call <vilib>:"Unset Busy.vi"() -> ()  [unwired: 11 in, 1 out]
          }
        }
      }
      frame "Test" {
        n170 = in-place {
          in-place-border: w415 -> [w427]
          in-place-border: [w422] -> w409
          n171 = in-place-cluster #4(w412) -> ("repository"=w417:refnum<class "SystemConfigRepo.lvclass">, "root"=w424:T3)
          n172 = call-dynamic "ReadTree.vi"("error in"=w427, "root"=w424, "repository in"=w417) -> ("error out"=w423:errorcluster, "repository out"=w419:refnum<class "NISE_CEF_Repository.lvclass">)  [unwired: 7 in]
          n173 = To More Specific Class(target class=w417, reference=w419, error in=w423) -> (specific class reference=w418:refnum<class "SystemConfigRepo.lvclass">, error out=w420:errorcluster)
          n174 = call-dynamic "WriteTree.vi"("error in"=w420, "repository in"=w418) -> ("error out"=w426:errorcluster, "root"=w425:T3, "repository out"=w421:refnum<class "NISE_CEF_Repository.lvclass">)  [unwired: 7 in]
          n175 = To More Specific Class(target class=w417, reference=w421, error in=w426) -> (specific class reference=w416:refnum<class "SystemConfigRepo.lvclass">, error out=w422:errorcluster)
          n176 = in-place-cluster #4("repository"=w416, "root"=w425) -> (w411:T2)
        }
        n177 = call <vilib>:"Send Local Message.vi"("message queue in"=w413, "message name"="PopulateTree", "error in"=w409) -> ("error out"=w414:errorcluster)  [unwired: 10 in, 2 out]
      }
      frame "HandleMenu" {
        n178 = Unflatten From String(type=T15 {"node id"="", "RightClickPath"=""} ("input cluster"), binary string=w446, error in (no error)=w447) -> (value=w444:T15, error out=w443:errorcluster)  [unwired: 2 in, 1 out]
        n179 = Unbundle By Name(w444) -> ("RightClickPath"=w439:string, "node id"=w442:string)
        n180 = call <vilib>:"IDtoNode.vi"("error in"=w443, "ID"=w442) -> ("error out"=w441:errorcluster, "node ref"=w428:T3)  [unwired: 7 in, 1 out]
        n181 = in-place {
          in-place-border: w441 -> [w465]
          in-place-border: [w462] -> w434
          in-place-border: [w461] -> w440
          in-place-border: w439 -> [w460]
          in-place-border: [w460] -> w438
          in-place-border: w437 -> [w459]
          in-place-border: w436 -> [w458]
          in-place-border: [w455] -> w430
          in-place-border: w428 -> [w454]
          n182 = in-place-dvr #5(w428) -> (w456:refnum<class "NISE_CEF_Node.lvclass">, w464:errorcluster)
          n183 = Merge Errors(w465, w464) -> (w463:errorcluster)
          n184 = call-dynamic "MenuHandler.vi"("tree control"=w458, "self reference"=w454, "main message queue"=w459, "error in"=w463, "menu string"=w460, "NISE_CEF_Node in"=w456) -> ("error out"=w462:errorcluster, "Unhandled"=w461:bool, "NISE_CEF_Node out"=w457:refnum<class "NISE_CEF_Node.lvclass">)  [unwired: 3 in]
          n185 = Not Equal?(x=w456, y=w457) -> (x != y?=w455:bool)
          n186 = in-place-dvr #5(w457) -> ()  [unwired: 2 out]
        }
        n187 = Unbundle By Name(w433) -> ("unsaved changes"=w431:bool)
        n188 = case shown="True" w440 {
          tunnel: w438 -> [_ w449]
          tunnel: [w448 w451] -> w435
          tunnel: w434 -> [w448 w450]
          frame False {
          }
          frame True {
            n189 = call <vilib>:"error generator.vi"("error in"=w450, "source"="configuration tool main.vi", "append error message"=w449, "error code (0)"=538506) -> ("error out"=w451:errorcluster)  [unwired: 5 in]
          }
        }
        n190 = Or(x=w431, y=w430) -> (x .or. y?=w429:bool)
        n191 = Bundle By Name(cluster=w433, "unsaved changes"=w429) -> (w432:T2)
      }
      frame "Script Include VI" {
        n192 = call "call include vi script.vi"("error in (no error)"=w467, "state cluster"=w468) -> ("error out"=w466:errorcluster)  [unwired: 9 in]
      }
      frame "-------TreeControl Operations-----------" {
        # "Dummy case to add a seperation in the Case Structure menu"
      }
      frame "AddNode" {
        n193 = call <vilib>:"Set Busy.vi"() -> ("error out"=w478:errorcluster)  [unwired: 10 in, 1 out]
        n194 = flat-sequence {
          tunnel: w497 -> [w499]
          tunnel: [w499] -> w484
          tunnel: w478 -> [_]
          frame #0 {
          }
        }
        n195 = Unflatten From String(type=T16 {"node type"="", "to add to"=""} ("input cluster"), binary string=w498) -> (value=w492:T16)  [unwired: 3 in, 2 out]
        n196 = Unbundle By Name(w492) -> ("to add to"=w490:string, "node type"=w487:string)
        n197 = in-place {
          in-place-border: w487 -> [w505]
          in-place-border: [w502] -> w486
          in-place-border: w484 -> [w501]
          in-place-border: [w500] -> w485
          n198 = in-place-cluster #6(w496) -> ("repository"=w504:refnum<class "SystemConfigRepo.lvclass">)
          n199 = call-dynamic "GetClassPath.vi"("error in"=w501, "class name"=w505, "Repository in"=w504) -> ("error out"=w500:errorcluster, "class path"=w502:path, "Repository out"=w503:refnum<class "SystemConfigRepo.lvclass">)  [unwired: 6 in]
          n200 = in-place-cluster #6("repository"=w503) -> (w480:T2)
        }
        n201 = Unbundle By Name(w480) -> ("glyph manager"=w472:T11)
        n202 = call <vilib>:"Get LV Class Default Value.vi"("error in (no error)"=w485, "class path"=w486) -> ("error out"=w494:errorcluster, "object"=w495:refnum<class>)  [unwired: 8 in]
        n203 = To More Specific Class(target class=refnum<class "NISE_CEF_Node.lvclass"> refnum ("NISE_CEF_Node.lvclass"), reference=w495, error in=w494) -> (specific class reference=w475:refnum<class "NISE_CEF_Node.lvclass">, error out=w476:errorcluster)
        n204 = call-dynamic "AddGlyphtoGManager.vi"("error in"=w476, "glyph manager"=w472, "NISE_CEF_Node in"=w475) -> ("error out"=w473:errorcluster, "glyph manager out"=w471:T11, "NISE_CEF_Node out"=w474:refnum<class "NISE_CEF_Node.lvclass">)  [unwired: 6 in]
        n205 = call <vilib>:"AddNode.vi"("error in"=w473, "node in"=w474, "parent node ID"=w490) -> ("error out"=w489:errorcluster, "summary"=w488:T25[])  [unwired: 7 in]
        n206 = call <vilib>:"PopulateTreeSumaryWithGlyphManager.vi"("error in"=w489, "glyph manager"=w471, "summary"=w488, "tree ref in"=w483) -> ("error out"=w479:errorcluster, "glyph manager out"=w477:T11)  [unwired: 6 in]
        n207 = Bundle By Name(cluster=w480, "unsaved changes"=TRUE, "glyph manager"=w477) -> (w482:T2)
        n208 = flat-sequence {
          tunnel: w479 -> [_]
          frame #0 {
            n209 = call <vilib>:"Unset Busy.vi"() -> ()  [unwired: 11 in, 1 out]
          }
        }
      }
      frame "Duplicate" {
        n210 = Unbundle By Name(w508) -> ("glyph manager"=w507:T11)
        n211 = call <vilib>:"IDtoNode.vi"("error in"=w515, "ID"=w516) -> ("error out"=w513:errorcluster, "invalid Id"=w512:bool, "node ref"=w514:T3)  [unwired: 7 in]
        n212 = case shown="False" w512 {
          tunnel: [w529 w531] -> w517
          tunnel: w514 -> [w528 _]
          tunnel: w513 -> [w525 w531]
          tunnel: w511 -> [w521 _]
          tunnel: w507 -> [w519 w530]
          tunnel: [w520 w530] -> w506
          frame False {
            n213 = call <vilib>:"DuplicateNode.vi"("same parent?"=TRUE ("s"), "error in"=w525, "node ref in"=w528) -> ("error out"=w526:errorcluster, "new node ref"=w527:T3)  [unwired: 7 in]
            n214 = call <vilib>:"SummaryWithGlyphManager.vi"("error in"=w526, "glyph manager"=w519, "node self ref"=w527) -> ("error out"=w523:errorcluster, "glyph manager out"=w518:T11, "summary"=w522:T25[])  [unwired: 6 in]
            n215 = call <vilib>:"PopulateTreeSumaryWithGlyphManager.vi"("error in"=w523, "glyph manager"=w518, "summary"=w522, "tree ref in"=w521) -> ("error out"=w529:errorcluster, "glyph manager out"=w520:T11)  [unwired: 6 in]
          }
          frame True {
          }
        }
        n216 = Bundle By Name(cluster=w508, "unsaved changes"=TRUE, "glyph manager"=w506) -> (w510:T2)
      }
      frame "RefreshNode" {
        # "Refreshes the node in the Tree               Sets the save flag to true                       This case can be called from the UIs of the nodes"
        n217 = Unbundle By Name(w534) -> ("glyph manager"=w533:T11)
        n218 = call <vilib>:"IDtoNode.vi"("error in"=w540, "ID"=w539) -> ("error out"=w538:errorcluster, "invalid Id"=w536:bool, "node ref"=w537:T3)  [unwired: 7 in]
        n219 = case shown="False" w536 {
          tunnel: [w551 w553] -> w542
          tunnel: w538 -> [w548 w553]
          tunnel: w537 -> [w547 _]
          tunnel: w535 -> [w546 _]
          tunnel: w533 -> [w544 w552]
          tunnel: [w545 w552] -> w532
          frame False {
            n220 = call <vilib>:"SummaryWithGlyphManager.vi"("error in"=w548, "glyph manager"=w544, "node self ref"=w547) -> ("error out"=w550:errorcluster, "glyph manager out"=w543:T11, "summary"=w549:T25[])  [unwired: 6 in]
            n221 = call <vilib>:"RefreshSubTreeWithGlyphManager.vi"("error in"=w550, "glyph manager"=w543, "node information"=w549, "tree ref in"=w546) -> ("error out"=w551:errorcluster, "glyph manager out"=w545:T11)  [unwired: 5 in, 1 out]
          }
          frame True {
          }
        }
        n222 = Bundle By Name(cluster=w534, "glyph manager"=w532) -> (w541:T2)
      }
      frame "SetDirtyDot" {
        n223 = Bundle By Name(cluster=w557, "unsaved changes"=TRUE ("SaveFlag")) -> (w556:T2)
      }
      frame "RemoveNode" {
        n224 = Unbundle By Name(w561) -> ("standard events"=w560:T5)
        n225 = call <vilib>:"IDtoNode.vi"("error in"=w568, "ID"=w569) -> ("error out"=w566:errorcluster, "invalid Id"=w564:bool, "node ref"=w565:T3)  [unwired: 7 in]
        n226 = case shown="False" w564 {
          tunnel: w566 -> [w577 w587]
          tunnel: w565 -> [w575 _]
          tunnel: [w579 w587] -> w567
          tunnel: w563 -> [w578 _]
          tunnel: w562 -> [w574 _]
          tunnel: w560 -> [w573 _]
          frame False {
            n227 = call "check if subpanel should be closed.vi"("error in"=w577, "SubPanel in"=w574, "node in"=w575) -> ("error out"=w572:errorcluster, "needs closing"=w570:bool, "node out"=w576:T3)  [unwired: 6 in]
            n228 = case shown="True" w570 {
              tunnel: w574 -> [_ w586]
              tunnel: w573 -> [_ w583]
              tunnel: w572 -> [w582 w585]
              tunnel: [w582 w584] -> w571
              frame False {
              }
              frame True {
                n229 = call "Remove UI without races.vi"("error in"=w585, "standard events"=w583, "sub panel ref in"=w586) -> ("error out"=w584:errorcluster)  [unwired: 7 in, 1 out]
              }
            }
            n230 = call <vilib>:"RemoveNode.vi"("error in"=w571, "node"=w576) -> ("error out"=w580:errorcluster, "node ID"=w581:string)  [unwired: 8 in]
            n231 = call <vilib>:"ClearTreeNode.vi"("error in"=w580, "tag"=w581, "tree reference"=w578) -> ("error out"=w579:errorcluster)  [unwired: 8 in]
          }
          frame True {
          }
        }
        n232 = Bundle By Name(cluster=w561, "unsaved changes"=TRUE) -> (w559:T2)
      }
      frame "PopulateTree" {
        n233 = Unbundle By Name(w607) -> ("current path"=w596:path, "glyph manager"=w589:T11, "root"=w604:T3)
        n234 = call <vilib>:"SummaryWithGlyphManager.vi"("error in"=w602, "glyph manager"=w589, "depth"=0 ("Depth"), "node self ref"=w604) -> ("error out"=w605:errorcluster, "glyph manager out"=w588:T11, "summary"=w606:T25[])  [unwired: 5 in]
        n235 = call <vilib>:"Check if File or Folder Exists.vi"("path"=w596) -> ("file or folder exists?"=w592:bool, "dup path"=w595:path)  [unwired: 8 in, 1 out]
        n236 = call <vilib>:"RefreshEntireTreeWithGlyphManager.vi"("calling VI in"=w598, "error in"=w605, "glyph manager"=w588, "array"=w606, "tree ref in"=w601) -> ("error out"=w600:errorcluster, "glyph manager out"=w590:T11)  [unwired: 5 in]
        n237 = Strip Path(path=w595) -> (name=w594:string)  [unwired: 1 out]
        n238 = Select(t=w594, s=w592, f="Tag Bus Configuration editor") -> (s? t:f=w593:string)
        n239 = Bundle By Name(cluster=w607, "glyph manager"=w590) -> (w591:T2)
        n240 = property class="VI"(reference=w598, error in=w600, "Front Panel.Title"=w593) -> (error out=w599:errorcluster)  [unwired: 1 out]
      }
      frame "CleansubPanel" {
        n241 = Unbundle By Name(w611) -> ("standard events"=w608:T5)
        n242 = call "Remove UI without races.vi"("error in"=w612, "standard events"=w608, "sub panel ref in"=w609) -> ("error out"=w610:errorcluster)  [unwired: 7 in, 1 out]
      }
      frame "ActivateNode" {
        n243 = Unbundle By Name(w620) -> ("standard events"=w617:T5)
        n244 = call <vilib>:"Set Busy.vi"("error in (no error)"=w623) -> ("error out"=w615:errorcluster)  [unwired: 9 in, 1 out]
        n245 = call <vilib>:"IDtoNode.vi"("error in"=w615, "ID"=w624) -> ("error out"=w616:errorcluster, "invalid Id"=w619:bool, "node ref"=w618:T3)  [unwired: 7 in]
        n246 = case shown="False" w619 {
          tunnel: w618 -> [w631 _]
          tunnel: [w632 w635] -> w614
          tunnel: w616 -> [w629 w636]
          tunnel: w621 -> [w628 _]
          tunnel: w617 -> [w625 w633]
          tunnel: w613 -> [w626 w634]
          frame False {
            n247 = call "Remove UI without races.vi"("error in"=w629, "standard events"=w625, "sub panel ref in"=w626) -> ("error out"=w630:errorcluster, "sub panel ref out"=w627:refnum<vi>)  [unwired: 7 in]
            n248 = call <vilib>:"LoadNodeUIStandardEvents.vi"("user event out"=w625, "error in"=w630, "sub panel ref in"=w627, "main queue"=w628, "node"=w631) -> ("error out"=w632:errorcluster)  [unwired: 6 in]
          }
          frame True {
            n249 = call "Remove UI without races.vi"("error in"=w636, "standard events"=w633, "sub panel ref in"=w634) -> ("error out"=w635:errorcluster)  [unwired: 7 in, 1 out]
          }
        }
        n250 = call <vilib>:"Unset Busy.vi"("error in (no error)"=w614) -> ("error out"=w622:errorcluster)  [unwired: 10 in]
      }
      frame "Move" {
        n251 = Unflatten From String(type=T17 {"node ref"=refnum, "new parent"=refnum} ("Cluster"), binary string=w649, error in (no error)=w648) -> (value=w644:T17, error out=w643:errorcluster)  [unwired: 2 in, 1 out]
        n252 = Unbundle By Name(w644) -> ("node ref"=w640:T3, "new parent"=w639:T3)
        n253 = call <vilib>:"MoveNode.vi"("error in"=w643, "new parent"=w639, "node"=w640) -> ("error out"=w641:errorcluster)  [unwired: 8 in]
        n254 = call <vilib>:"Send Local Message.vi"("message queue in"=w646, "message name"="PopulateTree", "error in"=w641) -> ("error out"=w647:errorcluster)  [unwired: 10 in, 2 out]
        n255 = Bundle By Name(cluster=w650, "unsaved changes"=TRUE) -> (w638:T2)
      }
      frame "RefreshNodeView" {
        # "This user event is used by editor nodes to update their subpanels when data in the tree changes."
        n256 = Unbundle By Name(w654) -> ("standard events.refresh UI"=w652:T9)
        n257 = Generate User Event(user event=w652, event data cluster=TRUE ("event data"), error in=w655) -> (error out=w653:errorcluster)  [unwired: 1 in, 1 out]
      }
      frame "NodeDataChange" {
        n258 = call <vilib>:"Send Local Message.vi"("message queue in"=w659, "message name"="RefreshNode", "message value"=w658, "error in"=w661) -> ("error out"=w660:errorcluster)  [unwired: 9 in, 2 out]
        n259 = Bundle By Name(cluster=w663, "unsaved changes"=TRUE) -> (w657:T2)
      }
    }
  }
  n260 = while "User Interface Event Handler" {
    tunnel: w20 -> [w670]
    tunnel: w7 -> [w666]
    tunnel: w5 -> [w665]
    tunnel: [w664] -> w3
    stop <- w669 stop-if-true
    n261 = event shown="[2] \"View\": Shortcut Menu Selection (User)" {
      selector: w665 -> [_ _ _ _ _ _ _ _ _ _]
      dyn-events: [_ _ _ _ _ _ _ _ _ _] -> w664
      timeout: _ -> [_ _ _ _ _ _ _ _ _ _]
      tunnel: w670 -> [w678 w697 w709 w751 w791 w798 w825 w829 w839 w844]
      tunnel: [_ _ _ _ TRUE _ _ _ _ _] -> w669
      tunnel: [w678 w696 w701 w753 w787 w798 w822 w829 w837 w843] -> w668
      tunnel: [w673 _ w702 w752 w788 w794 w821 w826 w835 w841] -> w667
      tunnel: w666 -> [w677 _ w707 w750 w789 w797 w820 w828 w836 w842]
      event "View": Shortcut Menu Activation? {
        n262 = event-data() -> ("CtlRef"=w684:refnum<vi>, "Coords"=w683:T26, "MenuRef"=w680:refnum<k9>)  [unwired: 1 in]
        n263 = invoke class="Tree (strict)" method="Point To Row Column"(reference=w684, error in=w677, "Point"=w683) -> (error out=w676:errorcluster, "Tag"=w682:string)  [unwired: 5 in, 6 out]
        n264 = call <vilib>:"IDtoNode.vi"("error in"=w676, "ID"=w682) -> ("error out"=w674:errorcluster, "invalid Id"=w679:bool, "node ref"=w681:T3)  [unwired: 7 in]
        n265 = case shown="False" w679 {
          selector: w679 -> [_ w694]
          tunnel: w681 -> [w688 _]
          tunnel: w680 -> [w687 _]
          tunnel: [w686 _] -> w675
          tunnel: [w685 _] -> w672
          tunnel: [_ w694] -> w671
          frame False {
            n266 = in-place {
              in-place-border: w687 -> [w691]
              in-place-border: [w689] -> w686
              n267 = in-place-dvr #7(w688) -> (w693:refnum<class "NISE_CEF_Node.lvclass">, w690:errorcluster)
              n268 = call-dynamic "ShortcutMenu.vi"("error in"=w690, "menu ref in"=w691, "node in"=w693) -> ("error out"=w689:errorcluster, "node out"=w692:refnum<class "NISE_CEF_Node.lvclass">)  [unwired: 6 in, 1 out]
              n269 = in-place-dvr #7(w692) -> (w685:errorcluster)  [unwired: 1 out]
            }
          }
          frame True {
          }
        }
        n270 = Merge Errors(w672, w675, w674) -> (w673:errorcluster)
        n271 = event-data("Discard?"=w671) -> ()  [unwired: 1 in, 1 out]
      }
      event User Event {
        n272 = event-data() -> ("node ref"=w699:T3)  [unwired: 1 in]
        n273 = call <vilib>:"NodetoID.vi"("node ref"=w699) -> ("ID"=w695:string)  [unwired: 9 in, 1 out]
        n274 = call <vilib>:"Send Local Message.vi"("message queue in"=w697, "message name"="NodeDataChange", "message value"=w695) -> ("message queue out"=w696:T13)  [unwired: 10 in, 2 out]
      }
      event "View": Shortcut Menu Selection (User) {
        # "=nodeID"
        n275 = event-data() -> ("ItemPath"=w705:string, "CtlRef"=w712:refnum<vi>, "Coords"=w713:T26)  [unwired: 1 in]
        n276 = invoke class="Tree (strict)" method="Point To Row Column"(reference=w712, error in=w707, "Point"=w713) -> (error out=w706:errorcluster, "Tag"=w708:string)  [unwired: 5 in, 6 out]
        n277 = Match Pattern(string=w705, regular expression=":") -> (before substring=w711:string, after substring=w710:string)  [unwired: 1 in, 2 out]
        n278 = case shown="Default" w711 {
          tunnel: w710 -> [_ _ _ w742]
          tunnel: w709 -> [w720 w731 w737 w744]
          tunnel: w708 -> [w718 w725 w735 w743]
          tunnel: [w717 w729 w734 w740] -> w704
          tunnel: [w716 w728 w732 w738] -> w703
          tunnel: w706 -> [w715 w724 w733 w739]
          tunnel: w705 -> [_ w721 _ _]
          frame "Remove" {
            n279 = call <vilib>:"Send Local Message.vi"("message queue in"=w720, "message name"="RemoveNode" ("Message Name"), "message value"=w718, "error in"=w715) -> ("message queue out"=w717:T13, "error out"=w716:errorcluster)  [unwired: 9 in, 1 out]
          }
          frame Default {
            n280 = Bundle By Name(cluster=T15 {"node id"="", "RightClickPath"=""} ("input cluster"), "node id"=w725, "RightClickPath"=w721) -> (w726:T15)
            n281 = Flatten To String(anything=w726, error in (no error)=w724) -> (data string=w722:string, error out=w723:errorcluster)  [unwired: 2 in, 1 out]
            n282 = call <vilib>:"Send Local Message.vi"("message queue in"=w731, "message name"="HandleMenu" ("Message Name"), "message value"=w722, "error in"=w723) -> ("message queue out"=w729:T13, "error out"=w728:errorcluster)  [unwired: 9 in, 1 out]
          }
          frame "Duplicate" {
            n283 = call <vilib>:"Send Local Message.vi"("message queue in"=w737, "message name"="Duplicate" ("Message Name"), "message value"=w735, "error in"=w733) -> ("message queue out"=w734:T13, "error out"=w732:errorcluster)  [unwired: 9 in, 1 out]
          }
          frame "Add" {
            n284 = Bundle By Name(cluster=T16 {"node type"="", "to add to"=""} ("input cluster"), "node type"=w742, "to add to"=w743) -> (w745:T16)
            n285 = Flatten To String(anything=w745) -> (data string=w746:string)  [unwired: 3 in, 2 out]
            n286 = call <vilib>:"Send Local Message.vi"("message queue in"=w744, "message name"="AddNode" ("Message Name"), "message value"=w746, "error in"=w739) -> ("message queue out"=w740:T13, "error out"=w738:errorcluster)  [unwired: 9 in, 1 out]
          }
        }
        n287 = call <vilib>:"Send Local Message.vi"("message queue in"=w704, "message name"="RefreshNodeView", "error in"=w703) -> ("message queue out"=w701:T13, "error out"=w702:errorcluster)  [unwired: 10 in, 1 out]
      }
      event "View": Drop {
        n288 = event-data() -> ("CtlRef"=w749:refnum<vi>, "Coords"=w748:T26)  [unwired: 1 in]
        n289 = invoke class="Tree (strict)" method="Point To Row Column"(reference=w749, error in=w750, "Point"=w748) -> (reference out=w767:refnum<vi>, error out=w766:errorcluster, "Tag"=w763:string)  [unwired: 5 in, 5 out]
        n290 = call <vilib>:"ValidDragDrop.vi"("error in"=w766, "drag over"=w763, "tree ref in"=w767) -> ("error out"=w758:errorcluster, "accepted"=w761:bool, "drag"=w765:string, "tree ref out"=w768:refnum<vi>)  [unwired: 5 in]
        n291 = call <vilib>:"IDtoNode.vi"("error in"=w758, "ID"=w763) -> ("error out"=w759:errorcluster, "invalid Id"=w756:bool, "node ref"=w762:T3)  [unwired: 7 in]
        n292 = call <vilib>:"IDtoNode.vi"("error in"=w759, "ID"=w765) -> ("error out"=w757:errorcluster, "invalid Id"=w755:bool, "node ref"=w764:T3)  [unwired: 7 in]
        n293 = Compound Arithmetic op=AND(w761, invert w756, invert w755) -> (w760:bool)
        n294 = case shown="True" w760 {
          tunnel: w765 -> [_ w784]
          tunnel: w768 -> [_ w786]
          tunnel: [_ TRUE] -> w754
          tunnel: w763 -> [_ w782]
          tunnel: w751 -> [w770 w771]
          tunnel: [w770 w778] -> w753
          tunnel: [w769 w777] -> w752
          tunnel: w764 -> [_ w773]
          tunnel: w762 -> [_ w772]
          tunnel: w757 -> [w769 w774]
          frame False {
          }
          frame True {
            n295 = invoke class="Tree (strict)" method="Edit Tree Items.Move Item"(reference=w786, error in=w774, "tag"=w784, "New Parent"=w782) -> (error out=w775:errorcluster)  [unwired: 3 in, 6 out]
            n296 = Bundle By Name(cluster=T17 {"node ref"=refnum, "new parent"=refnum} ("Cluster"), "new parent"=w772, "node ref"=w773) -> (w781:T17)
            n297 = Flatten To String(anything=w781, error in (no error)=w775) -> (data string=w780:string, error out=w776:errorcluster)  [unwired: 2 in, 1 out]
            n298 = call <vilib>:"Send Local Message.vi"("message queue in"=w771, "message name"="Move", "message value"=w780, "error in"=w776) -> ("message queue out"=w778:T13, "error out"=w777:errorcluster)  [unwired: 9 in, 1 out]
          }
        }
        n299 = event-data("Accepted?"=w754) -> ()  [unwired: 1 in, 1 out]
      }
      event "Exit": Value Change {
        # "Exit the application                                           >> Stop this message generator loop    Cleaning errors if the other loop stop this one"
        n300 = event-data() -> ()  [unwired: 1 in, 1 out]
        n301 = call <vilib>:"Send Local Message.vi"("message queue in"=w791, "message name"="Close", "error in"=w789) -> ("message queue out"=w787:T13, "error out"=w792:errorcluster)  [unwired: 10 in, 1 out]
        n302 = call <vilib>:"Clear Errors.vi"("error in (no error)"=w792) -> ("error out"=w788:errorcluster)  [unwired: 6 in]
      }
      event "View": Drag Starting? {
        n303 = event-data() -> ("Data"=w804:T27, "CtlRef"=w806:refnum<vi>, "Coords"=w805:T26)  [unwired: 1 in]
        n304 = invoke class="Tree (strict)" method="Point To Row Column"(reference=w806, error in=w797, "Point"=w805) -> (error out=w796:errorcluster, "Tag"=w803:string)  [unwired: 5 in, 6 out]
        n305 = call <vilib>:"IDtoNode.vi"("error in"=w796, "ID"=w803) -> ("error out"=w795:errorcluster, "invalid Id"=w802:bool, "node ref"=w801:T3)  [unwired: 7 in]
        n306 = case shown="False" w802 {
          tunnel: w801 -> [w812 _]
          tunnel: [w809 TRUE ("Removable")] -> w799
          tunnel: w795 -> [w808 w818]
          tunnel: [w807 w818] -> w794
          frame False {
            n307 = in-place {
              in-place-border: [w815] -> w811
              in-place-border: w808 -> [w814]
              in-place-border: [w813] -> w807
              n308 = in-place-dvr #8(w812) -> (w817:refnum<class "NISE_CEF_Node.lvclass">)  [unwired: 1 out]
              n309 = call-dynamic "EditOptions.vi"("error in"=w814, "node in"=w817) -> ("error out"=w813:errorcluster, "edit options"=w815:T28, "node out"=w816:refnum<class "NISE_CEF_Node.lvclass">)  [unwired: 6 in, 1 out]
              n310 = in-place-dvr #8(w816) -> ()  [unwired: 2 out]
            }
            n311 = Unbundle By Name(w811) -> ("movable"=w810:bool)
            n312 = Not(x=w810) -> (.not. x?=w809:bool)
          }
          frame True {
          }
        }
        n313 = event-data("Data"=w804, "Drag Mode"=enum32{"copy or move", "copy only", "move only"}."move only", "Discard?"=w799) -> ()  [unwired: 1 in, 1 out]
      }
      event "View": Value Change {
        n314 = event-data() -> ("NewVal"=w823:string)  [unwired: 1 in]
        n315 = call <vilib>:"Send Local Message.vi"("message queue in"=w825, "message name"="ActivateNode" ("Message Name"), "message value"=w823, "error in"=w820) -> ("message queue out"=w822:T13, "error out"=w821:errorcluster)  [unwired: 9 in, 1 out]
      }
      event "View": event type 3.0.xa000003a {
        n316 = event-data() -> ("CtlRef"=w834:refnum<vi>, "Coords"=w831:T26)  [unwired: 1 in]
        n317 = invoke class="Tree (strict)" method="Point To Row Column"(reference=w834, error in=w828, "Point"=w831) -> (reference out=w833:refnum<vi>, error out=w827:errorcluster, "Tag"=w832:string)  [unwired: 5 in, 5 out]
        n318 = call <vilib>:"ValidDragDrop.vi"("error in"=w827, "drag over"=w832, "tree ref in"=w833) -> ("error out"=w826:errorcluster, "accepted"=w830:bool)  [unwired: 5 in, 2 out]
        n319 = event-data("Accepted?"=w830) -> ()  [unwired: 1 in, 1 out]
      }
      event Panel Close? {
        # "Intercepts the upper right close panel operation to allow a smooth shutdown as opposed to immediately killing the app."
        n320 = event-data() -> ()  [unwired: 1 in, 1 out]
        n321 = call <vilib>:"Send Local Message.vi"("message queue in"=w839, "message name"="Close?", "error in"=w836) -> ("message queue out"=w837:T13, "error out"=w835:errorcluster)  [unwired: 10 in, 1 out]
        n322 = event-data("Discard?"=TRUE) -> ()  [unwired: 1 in, 1 out]
      }
      event Menu Selection (User) {
        n323 = event-data() -> ("ItemPath"=w845:string)  [unwired: 1 in]
        n324 = case shown="\"_Tools:Script Include VI\"" w845 {
          tunnel: w844 -> [w847 w853 w858 w863 w868 w873 w882 w887 w892 w897 w902 w907 w913 w917]
          tunnel: [w847 w849 w854 w859 w864 w869 w879 w884 w889 w894 w899 w904 w910 w916] -> w843
          tunnel: w842 -> [w846 w851 w856 w861 w866 w871 w878 w885 w890 w895 w900 w905 w911 w915]
          tunnel: [w846 w850 w855 w860 w865 w870 w876 w883 w888 w893 w898 w903 w909 w914] -> w841
          frame Default {
            n325 = One Button Dialog(message="Unknown Menu Option") -> ()  [unwired: 1 in, 1 out]
          }
          frame "_File:_New" {
            n326 = call <vilib>:"Send Local Message.vi"("message queue in"=w853, "message name"="New?" ("Message Name"), "error in"=w851) -> ("message queue out"=w849:T13, "error out"=w850:errorcluster)  [unwired: 10 in, 1 out]
          }
          frame "_File:_Open" {
            n327 = call <vilib>:"Send Local Message.vi"("message queue in"=w858, "message name"="Open?" ("Message Name"), "error in"=w856) -> ("message queue out"=w854:T13, "error out"=w855:errorcluster)  [unwired: 10 in, 1 out]
          }
          frame "_File:_Save" {
            n328 = call <vilib>:"Send Local Message.vi"("message queue in"=w863, "message name"="Save" ("Message Name"), "error in"=w861) -> ("message queue out"=w859:T13, "error out"=w860:errorcluster)  [unwired: 10 in, 1 out]
          }
          frame "_File:Save As..." {
            n329 = call <vilib>:"Send Local Message.vi"("message queue in"=w868, "message name"="SaveAs" ("Message Name"), "error in"=w866) -> ("message queue out"=w864:T13, "error out"=w865:errorcluster)  [unwired: 10 in, 1 out]
          }
          frame "_File:_Exit" {
            n330 = call <vilib>:"Send Local Message.vi"("message queue in"=w873, "message name"="Close?" ("Message Name"), "error in"=w871) -> ("message queue out"=w869:T13, "error out"=w870:errorcluster)  [unwired: 10 in, 1 out]
          }
          frame "_Tools:Multiple Parameter Editor" {
            n331 = call <vilib>:"Send Local Message.vi"("message queue in"=w882, "message name"="CleansubPanel", "error in"=w878) -> ("message queue out"=w881:T13, "error out"=w877:errorcluster)  [unwired: 10 in, 1 out]
            n332 = call <vilib>:"Send Local Message.vi"("message queue in"=w881, "message name"="Custom View", "message value"="Multiple Parameter Editor" ("Message Name"), "error in"=w877) -> ("message queue out"=w879:T13, "error out"=w876:errorcluster)  [unwired: 9 in, 1 out]
          }
          frame "_Tools:Test" {
            n333 = call <vilib>:"Send Local Message.vi"("message queue in"=w887, "message name"="Test", "error in"=w885) -> ("message queue out"=w884:T13, "error out"=w883:errorcluster)  [unwired: 10 in, 1 out]
          }
          frame "_Tools:Deploy Tool" {
            n334 = call <vilib>:"Send Local Message.vi"("message queue in"=w892, "message name"="DeployTool", "error in"=w890) -> ("message queue out"=w889:T13, "error out"=w888:errorcluster)  [unwired: 10 in, 1 out]
          }
          frame "_Tools:Save Binary" {
            n335 = call <vilib>:"Send Local Message.vi"("message queue in"=w897, "message name"="Save Binary", "error in"=w895) -> ("message queue out"=w894:T13, "error out"=w893:errorcluster)  [unwired: 10 in, 1 out]
          }
          frame "_Tools:Script Include VI" {
            n336 = call <vilib>:"Send Local Message.vi"("message queue in"=w902, "message name"="Script Include VI", "error in"=w900) -> ("message queue out"=w899:T13, "error out"=w898:errorcluster)  [unwired: 10 in, 1 out]
          }
          frame "_Tools:Load Binary" {
            n337 = call <vilib>:"Send Local Message.vi"("message queue in"=w907, "message name"="Load Binary", "error in"=w905) -> ("message queue out"=w904:T13, "error out"=w903:errorcluster)  [unwired: 10 in, 1 out]
          }
          frame "_Tools:Refresh Plugins" {
            n338 = call <vilib>:"Send Local Message.vi"("message queue in"=w913, "message name"="FindPluginNodes", "message value"="Refresh", "error in"=w911) -> ("message queue out"=w910:T13, "error out"=w909:errorcluster)  [unwired: 9 in, 1 out]
          }
          frame "_Tools:Edit Plugin Search Paths" {
            n339 = call <vilib>:"Send Local Message.vi"("message queue in"=w917, "message name"="Edit Plugin Search Paths", "error in"=w915) -> ("message queue out"=w916:T13, "error out"=w914:errorcluster)  [unwired: 10 in, 1 out]
          }
        }
      }
    }
    n340 = call "send error message.vi"("error in"=w667, "message queue in"=w668) -> ()  [unwired: 9 in, 1 out]
  }
  n341 = Unregister For Events(event registration refnum=w3) -> ()  [unwired: 1 in, 1 out]
  n342 = call <vilib>:"DestroyStandardEvents.vi"("error in"=w2, "standard events"=w1) -> ()  [unwired: 9 in, 1 out]
